vi "TransformHelper.vi"(8 "error in (no error)":errorcluster, 9 "Multiplier":sgl, 10 "Power":sgl, 11 "Refnum in":T1) -> (0 "error out":errorcluster, 1 "Time, ms":u32, 3 "Refnum out":T1)   [LabVIEW 2023]
uses:
  <vilib>/vision/Image Controls.llb/IMAQ Image.ctl
  OpenCVWrapper/build/OpenCVWrapper.dll
panel:
  in  "Divider":dbl=100.0 format="%#_13g"
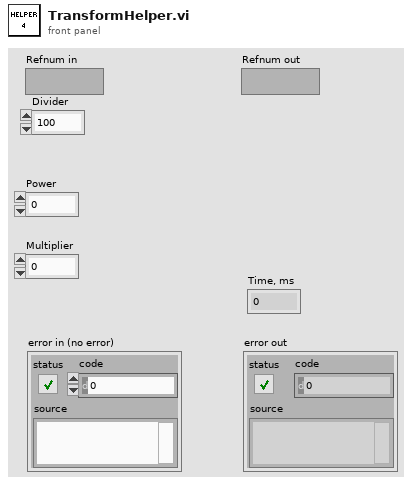
[diagram p1: front panel]
types:
  T1 = typedef "IMAQ Image.ctl" = refnum<image>
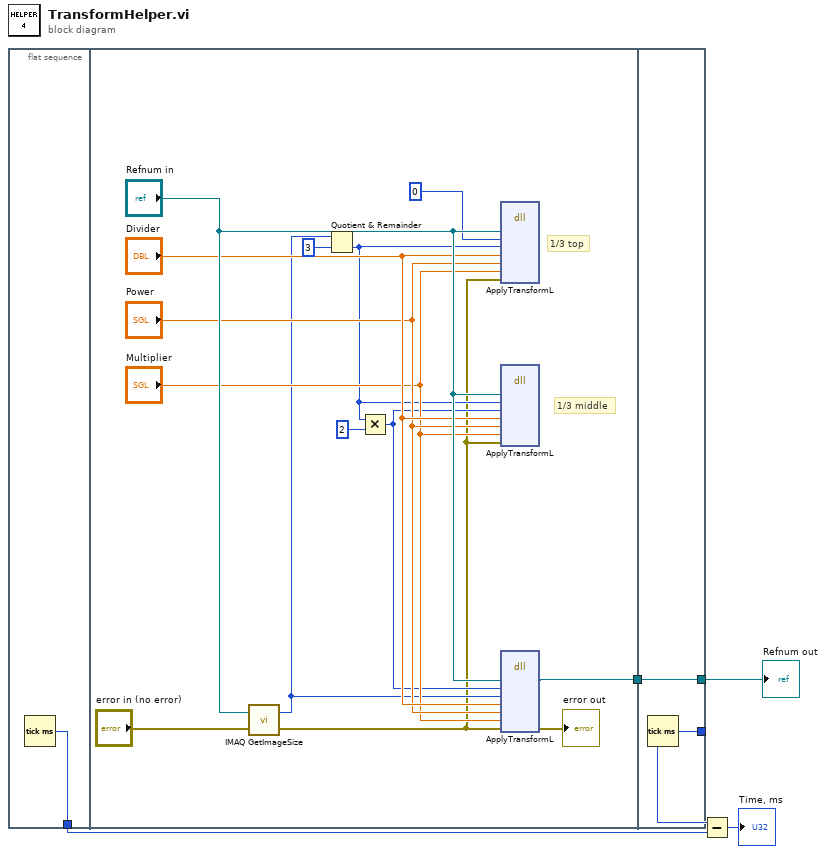
[diagram p0: block diagram]
diagram:
  n1 = flat-sequence {
    tunnel: [w6] -> w4
    tunnel: [w7] -> w1
    tunnel: [w22] -> w5
    tunnel: [w21] -> w2
    tunnel: w1 -> [w21]
    frame #0 {
      n2 = Tick Count (ms)() -> (millisecond timer value=w6:u32)
    }
    frame #1 {
      # "1/3 middle"
      # "1/3 top"
      n3 = call "IMAQ GetImageSize"("Image"="Refnum in", "error in (no error)"="error in (no error)") -> ("Y Resolution"=w10:i32, "error out"=w8:errorcluster)  [unwired: 2 in, 1 out]
      n4 = Quotient & Remainder(x=w10, y=3) -> (floor(x/y)=w13:i32)  [unwired: 1 out]
      n5 = Multiply(x=w13, y=2) -> (x*y=w11:i32)
      n6 = dll-call lib="C:/Users/Andrey/Desktop/xev - c leaned2/OpenCVWrapper/build/OpenCVWrapper.dll" fn="ApplyTransformL"("Src"="Refnum in", "StartLine"=0, "EndLine"=w13, "Divider"="Divider", "Power"="Power", "Multiplier"="Multiplier", "arg5"=w8) -> ()  [unwired: 11 in, 2 out]
      n7 = dll-call lib="C:/Users/Andrey/Desktop/xev - c leaned2/OpenCVWrapper/build/OpenCVWrapper.dll" fn="ApplyTransformL"("Src"="Refnum in", "StartLine"=w13, "EndLine"=w11, "Divider"="Divider", "Power"="Power", "Multiplier"="Multiplier", "arg5"=w8) -> ()  [unwired: 11 in, 2 out]
      n8 = dll-call lib="C:/Users/Andrey/Desktop/xev - c leaned2/OpenCVWrapper/build/OpenCVWrapper.dll" fn="ApplyTransformL"("Src"="Refnum in", "StartLine"=w11, "EndLine"=w10, "Divider"="Divider", "Power"="Power", "Multiplier"="Multiplier", "arg5"=w8) -> ("Src"=w7:T1, "arg5"=→"error out":errorcluster)  [unwired: 9 in, 2 out]
    }
    frame #2 {
      n9 = Tick Count (ms)() -> (millisecond timer value=w22:u32)
    }
  }
  n10 = Subtract(x=w5, y=w4) -> (x-y=→"Time, ms":u32)
  "Refnum out" <- w2
